vi "Get SMO Public API enum.vi"(8 "error in (no error)":errorcluster, 11 "Instrument.Framework-Template in":refnum<class "Instrument.Framework-Template.lvclass">) -> (0 "error out":errorcluster, 2 "Commands":variant, 3 "Instrument.Framework-Template out":refnum<class "Instrument.Framework-Template.lvclass">)   [LabVIEW 2019, in "Instrument.Framework-Template.lvclass"]
doc: "Override this VI to return a list of commands supported by your Instrument"
uses:
  Instrument.Framework-Template.lvclass
  Typedefs/Instrument.Framework-Template.Commands--Enum.ctl
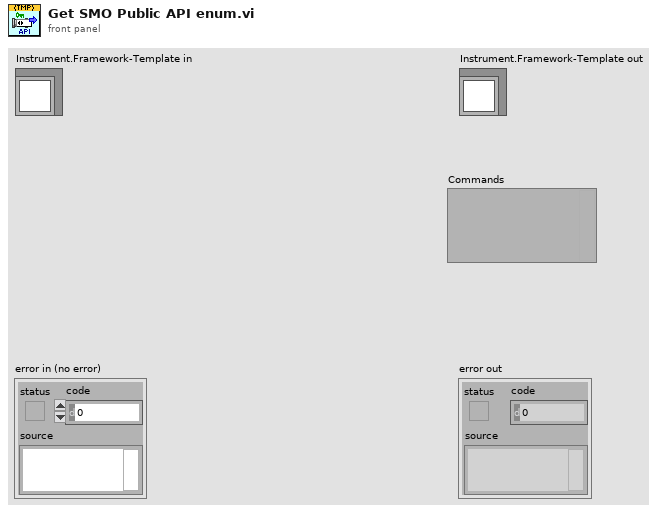
[diagram p1: front panel]
types:
  T1 = typedef "Instrument.Framework-Template.lvclass/Instrument.Framework-Template.Commands--Enum.ctl" = enum16{"Do Something"}
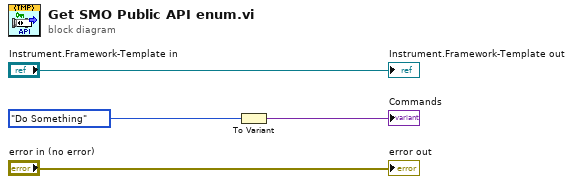
[diagram p0: block diagram]
diagram:
  n1 = To Variant(anything=Instrument.Framework-Template.Commands--Enum."Do Something" ("Commands")) -> (Variant=→"Commands":variant)
  "error out" <- "error in (no error)"
  "Instrument.Framework-Template out" <- "Instrument.Framework-Template in"
